vi "FlatToRichnixnet_grpc_StartRequest.vi"(5 "OutputClusterType":T1, 11 "InputCluster":T3) -> (3 "OutputCluster":T1)   [LabVIEW 2025, in "xnet-grpc_client.lvlib"]
uses:
  nixnet_grpc_StartRequest_Flat.ctl
  nidevice_grpc_Session_Flat.ctl
  nixnet_grpc_StartStopScope.ctl
  nixnet_grpc_StartRequest.ctl
  nixnet_grpc_StartRequest_scope_enum/nixnet_grpc_StartRequest_scope_enum.lvclass
  nidevice_grpc_Session.ctl
  xnet-grpc_client.lvlib
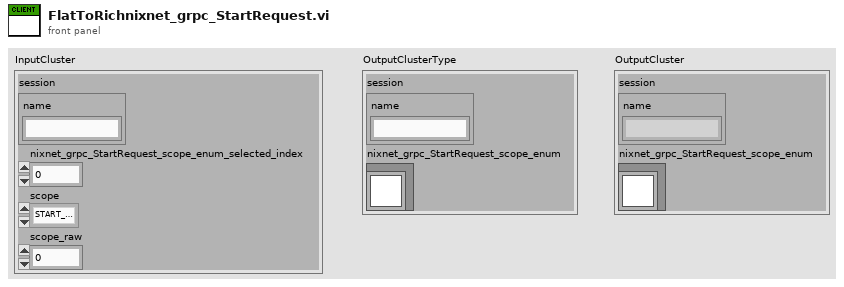
[diagram p1: front panel]
types:
  T1 = typedef "xnet-grpc_client.lvlib/nixnet_grpc_StartRequest.ctl" = cluster{"session":T2, "nixnet_grpc_StartRequest_scope_enum":refnum<class "nixnet_grpc_StartRequest_scope_enum.lvclass">}
  T2 = typedef "xnet-grpc_client.lvlib/nidevice_grpc_Session.ctl" = cluster{"name":string}
  T3 = typedef "xnet-grpc_client.lvlib/nixnet_grpc_StartRequest_Flat.ctl" = cluster{"session":T4, "nixnet_grpc_StartRequest_scope_enum_selected_index":i32, "scope":T5, "scope_raw":u32}
  T4 = typedef "xnet-grpc_client.lvlib/nidevice_grpc_Session_Flat.ctl" = cluster{"name":string}
  T5 = typedef "xnet-grpc_client.lvlib/nixnet_grpc_StartStopScope.ctl" = enum32{"START_STOP_SCOPE_NORMAL", "START_STOP_SCOPE_SESSION_ONLY", "START_STOP_SCOPE_INTERFACE_ONLY", "START_STOP_SCOPE_SESSION_ONLY_BLOCKING"}
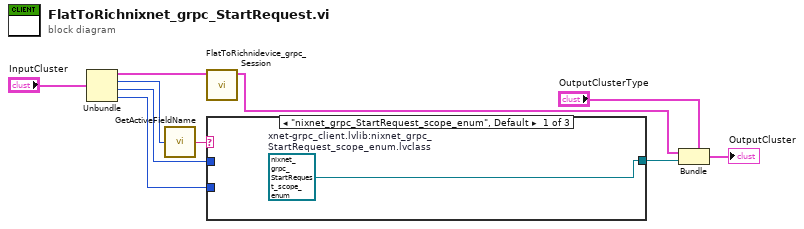
[diagram p0: block diagram]
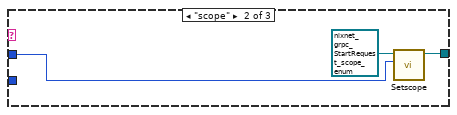
[diagram p2: hidden frame]
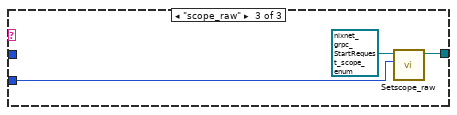
[diagram p3: hidden frame]
diagram:
  n1 = Unbundle "Unbundle"("InputCluster") -> ("session"=w7:T4, "nixnet_grpc_StartRequest_scope_enum_selected_index"=w5:i32, "scope"=w2:T5, "scope_raw"=w1:u32)
  n2 = call "GetActiveFieldName.vi"("protobuf index"=w5) -> ("oneof field name"=w4:string)
  n3 = call "FlatToRichnidevice_grpc_Session.vi"("InputCluster"=w7) -> ("OutputCluster"=w6:T2)  [unwired: 10 in]
  n4 = case "nixnet_grpc_StartRequest_scope_enum" shown="\"nixnet_grpc_StartRequest_scope_enum\", Default" w4 {
    tunnel: [w11 w13 w16] -> w3
    tunnel: w2 -> [_ w14 _]
    tunnel: w1 -> [_ _ w17]
    frame "nixnet_grpc_StartRequest_scope_enum", Default {
      w11 = refnum<class "nixnet_grpc_StartRequest_scope_enum.lvclass"> refnum  # xnet-grpc_client.lvlib:nixnet_grpc_StartRequest_scope_enum.lvclass
    }
    frame "scope" {
      n5 = call "Setscope.vi"("Set_Val"=w14, "OneOfTemplate in"=refnum<class "nixnet_grpc_StartRequest_scope_enum.lvclass"> refnum) -> ("OneOfTemplate out"=w13:refnum<class "nixnet_grpc_StartRequest_scope_enum.lvclass">)  [unwired: 8 in, 1 out]
    }
    frame "scope_raw" {
      n6 = call "Setscope_raw.vi"("Set_Val"=w17, "OneOfTemplate in"=refnum<class "nixnet_grpc_StartRequest_scope_enum.lvclass"> refnum) -> ("OneOfTemplate out"=w16:refnum<class "nixnet_grpc_StartRequest_scope_enum.lvclass">)  [unwired: 8 in, 1 out]
    }
  }
  n7 = Bundle "Bundle"(cluster="OutputClusterType", "session"=w6, "nixnet_grpc_StartRequest_scope_enum"=w3) -> (→"OutputCluster":T1)
